vi "passFail.vi"(11 "Boolean":bool) -> (3 "Result":T1)   [LabVIEW 2015]
uses:
  Typedefs/PassFailTest.ctl
  Typedefs/ILCBTTypedefs.lvlib
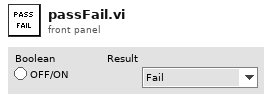
[diagram p1: front panel]
types:
  T1 = typedef "ILCBTTypedefs.lvlib/PassFailTest.ctl" = enum16{"Fail", "Pass", "NA"}
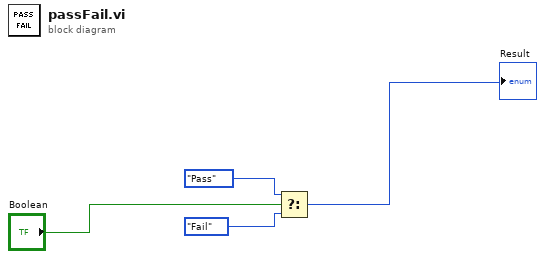
[diagram p0: block diagram]
diagram:
  n1 = Select(t=PassFailTest."Pass" ("Result"), s="Boolean", f=PassFailTest."Fail" ("Result")) -> (s? t:f=→"Result":T1)
